vi "get_cmd_string.vi"(10 "目标位置":dbl[](array[numeric]), 11 "目标取向":dbl[][](array[numeric])) -> (2 "length":i32, 3 "String":string)   [LabVIEW 2017]
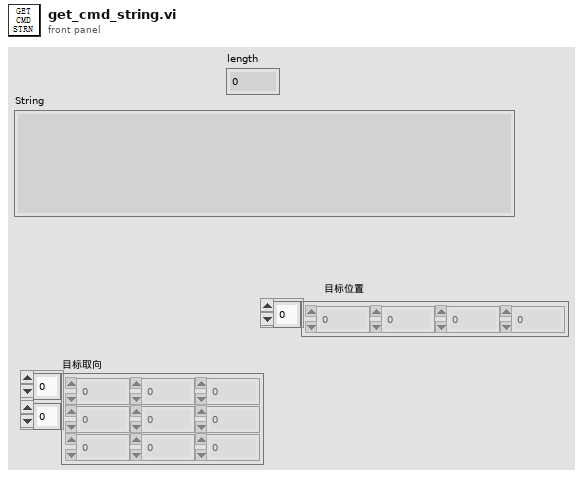
[diagram p1: front panel]
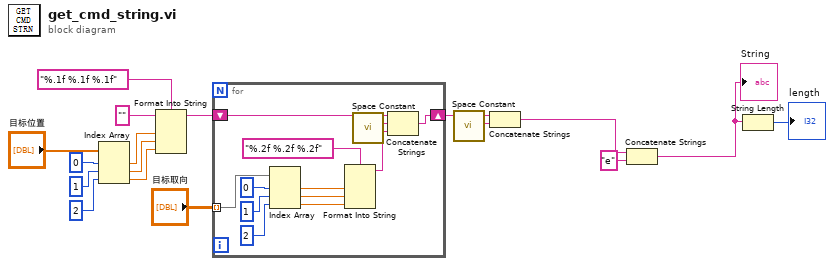
[diagram p0: block diagram]
diagram:
  n1 = Index Array(array="目标位置", index #1=0 ("index"), index #2=1 ("index"), index #3=2 ("index")) -> (element #1=w12:dbl, element #2=w11:dbl, element #3=w10:dbl)
  n2 = Format Into String(format string="%.1f %.1f %.1f", initial string="", w12, w11, w10) -> (resulting string=w7:string)  [unwired: 1 in, 1 out]
  n3 = for {
    tunnel: "目标取向" -> [w27] mode=indexing
    shift-right: [w28] -> w8
    shift-left: w7 -> [w29]
    n4 = Index Array(array=w27, index #1=0 ("index"), index #2=1 ("index"), index #3=2 ("index")) -> (element #1=w23:dbl, element #2=w22:dbl, element #3=w21:dbl)
    n5 = Format Into String(format string="%.2f %.2f %.2f", w23, w22, w21) -> (resulting string=w19:string)  [unwired: 2 in, 1 out]
    n6 = call <vilib>:"Space Constant.vi"() -> ("String"=w18:string)
    n7 = Concatenate Strings(w29, w18, w19) -> (w28:string)
  }
  n8 = call <vilib>:"Space Constant.vi"() -> ("String"=w5:string)
  n9 = Concatenate Strings(w8, w5) -> (w3:string)
  n10 = Concatenate Strings(w3, "e" ("string")) -> (w2:string)
  "String" <- w2
  n11 = String Length(string=w2) -> (length=→"length":i32)
